vi "Open Connection.vi"(11 "conninfo":string) -> (0 "error out":errorcluster, 2 "conn":u32, 3 "PQStatus":T1(ring))   [LabVIEW 2017]
uses:
  PostgreSQL2LabVIEW/libpqlv/libpqlv.lvlib
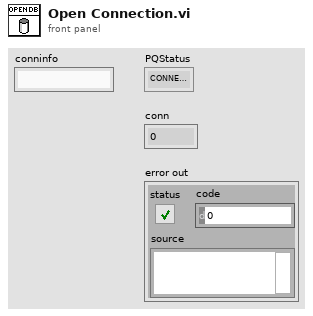
[diagram p1: front panel]
types:
  T1 = enum32{"CONNECTION_OK", "CONNECTION_BAD", "CONNECTION_STARTED", "CONNECTION_MADE", "CONNECTION_AWAITING_RESPONSE", "CONNECTION_AUTH_OK", "CONNECTION_SETENV", "CONNECTION_SSL_STARTUP", "CONNECTION_NEEDED"}
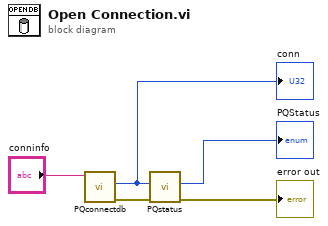
[diagram p0: block diagram]
diagram:
  n1 = call "PQconnectdb.vi"("conninfo"="conninfo") -> ("error out"=w2:errorcluster, "conn"=w5:u32)  [unwired: 9 in]
  "conn" <- w5
  n2 = call "PQstatus.vi"("error in (no error)"=w2, "conn"=w5) -> ("error out"=→"error out":errorcluster, "PQStatus"=→"PQStatus":T1)  [unwired: 8 in]
